vi "DeviceIsOpen.vi"(6 "Delay between send and receive [ms]":i32=100, 8 "error in (no error)":errorcluster, 11 "GenericDevice in":refnum<class "GenericDevice.lvclass">) -> (0 "error out":errorcluster, 1 "ID":i32, 2 "device is open?":bool, 3 "GenericDevice out":refnum<class "GenericDevice.lvclass">)   [LabVIEW 2023, in "GenericDevice.lvclass"]
doc: "Returns true if selected CCD is open."
uses:
  GenericDevice.lvclass
  IsOpen.ctl
  GenericDevice.lvclass/GenericDevice.ctl
  9c9fad9a-af94-4ee9-a58f-4085316ae059.vi
  c3d4486f-2ecf-46ea-b389-a9a9b166625e.vi
  0743153f-97fe-4723-9c7c-0ed28467d69b.vi
  <vilib>/JDP Science/JSONtext/Variant to JSON Text.vi
  <vilib>/JDP Science/JSONtext/Set Item.vi
  <vilib>/JDP Science/JSONtext/JSON text to Variant.vi
  <vilib>/JDP Science/JSONtext/LVClass Serializer/JSONtext LVClass Serializer.lvclass
panel:
  # "Connector Pane"
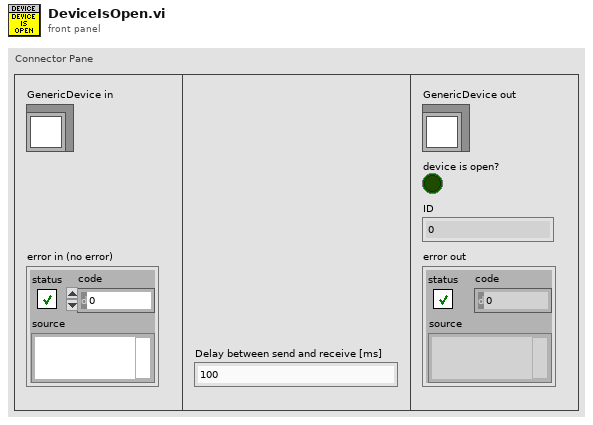
[diagram p1: front panel]
types:
  T1 = typedef "GenericDevice.lvclass/IsOpen.ctl" = cluster{"open":bool}
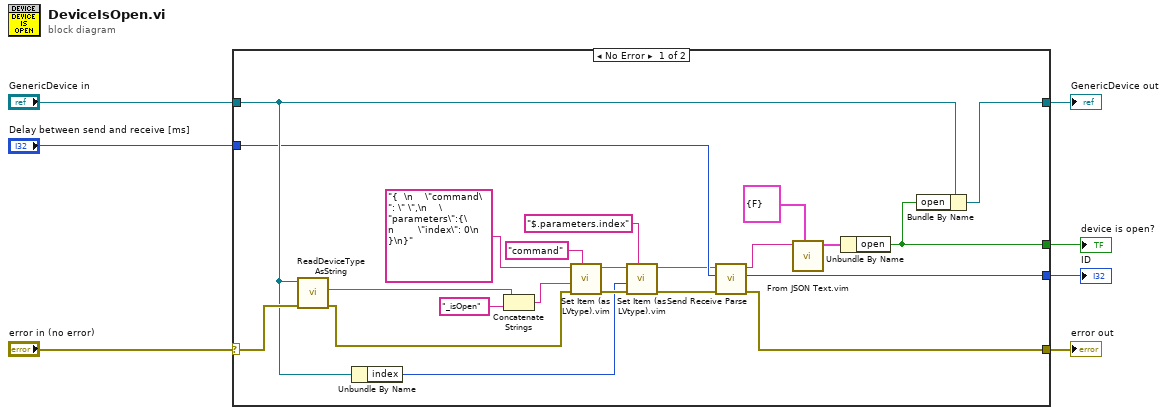
[diagram p0: block diagram]
diagram:
  n1 = case shown="No Error" "error in (no error)" {
    selector: "error in (no error)" -> [w13 w31]
    tunnel: [w16 w31] -> w6
    tunnel: [w17 w30] -> w4
    tunnel: "GenericDevice in" -> [w11 w30]
    tunnel: [w15 _] -> w3
    tunnel: [w14 _] -> w2
    tunnel: "Delay between send and receive [ms]" -> [w9 _]
    frame No Error {
      n2 = call "ReadDeviceTypeAsString.vi"("error in (no error)"=w13, "GenericDevice.lvclass"=w11) -> ("error out"=w12:errorcluster, "String"=w10:string)  [unwired: 7 in, 1 out]
      n3 = Unbundle By Name(w11) -> ("index"=w22:i32)
      n4 = Concatenate Strings(w10, "_isOpen" ("string")) -> (w23:string)
      n5 = call "Set Item (as LVtype).vim"("$Path or Item Name"="command", "error in (no error)"=w12, "Anything"=w23, "JSON"="{  \n    \"command\": \" \",\n    \"parameters\":{\n        \"index\": 0\n    }\n}") -> ("error out"=w27:errorcluster, "<JSON>"=w28:string)  [unwired: 4 in, 1 out]
      n6 = call "Set Item (as LVtype).vim"("$Path or Item Name"="$.parameters.index", "error in (no error)"=w27, "Anything"=w22, "JSON"=w28) -> ("error out"=w21:errorcluster, "<JSON>"=w8:string)  [unwired: 4 in, 1 out]
      n7 = call "Send Receive Parse.vi"("error in"=w21, "Delay between send and receive [ms]"=w9, "<JSON>"=w8) -> ("error out"=w16:errorcluster, "ID"=w14:i32, "results-JSON string"=w18:string)  [unwired: 6 in]
      n8 = call "From JSON Text.vim"("Data Type and Default Value"=T1 {"open"=FALSE} ("CCD open for communication?"), "JSON"=w18) -> ("Data out"=w19:T1)  [unwired: 8 in, 1 out]
      n9 = Unbundle By Name(w19) -> ("open"=w15:bool)
      n10 = Bundle By Name(cluster=w11, "open"=w15) -> (w17:refnum<class "GenericDevice.lvclass">)
    }
    frame Error {
    }
  }
  "error out" <- w6
  "GenericDevice out" <- w4
  "ID" <- w2
  "device is open?" <- w3
